vi "Read Drive Operation.vi"(8 "Command Info":T3) -> (0 "Command Info":T3, 1 "SubSystem Data":T1)   [LabVIEW 2017]
doc: "Returns the details about the currently executing command."
uses:
  Implementation/Drive Operations.ctl
  Implementation/Drive Setpoints.ctl
  <vilib>/Rock Robotics/WPI/Framework/Completion Status.ctl
  <vilib>/Rock Robotics/WPI/Framework/Completion Notifier.ctl
  <vilib>/Rock Robotics/WPI/Framework/Command Status Info.ctl
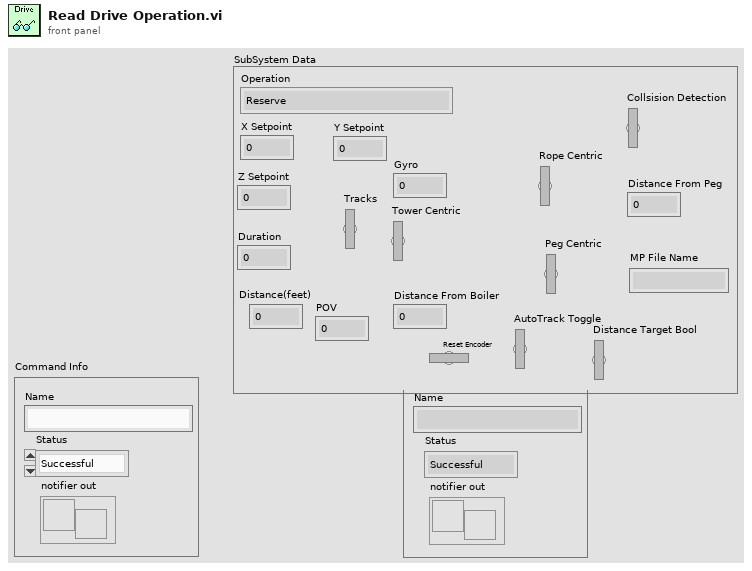
[diagram p1: front panel]
types:
  T1 = typedef "Drive Setpoints.ctl" = cluster{"Operation":T2, "X Setpoint":dbl, "Y Setpoint":dbl, "Duration":dbl, "Z Setpoint":dbl, "Tracks":bool, "Gyro":dbl, "Tower Centric":bool, "POV":i16, "Distance(feet)":dbl, "Distance From Boiler":dbl, "Peg Centric":bool, "Rope Centric":bool, "Distance Target Bool":bool, "AutoTrack Toggle":bool, "Collsision Detection":bool, "Distance From Peg":dbl, "Reset Encoder":bool, "MP File Name":string}
  T2 = typedef "Drive Operations.ctl" = enum16{"Reserve", "Motion Profiling", "Read Current", "Immediate Robot Centric", "Drive for Time Robot Centric", "Immediate Field Centric", "Drive For Time Field Centric", "Immediate MecaTrak", "Drive For Time MecaTrak", "Button Adjust", "Drive for Distance", "Drive Directional Immediate"}
  T3 = typedef "Command Status Info.ctl" = cluster{"Name":string, "Status":T4, "notifier out":T5}
  T4 = typedef "Completion Status.ctl" = enum16{"Successful", "Aborted", "Incomplete"}
  T5 = typedef "Completion Notifier.ctl" = refnum<notifier>
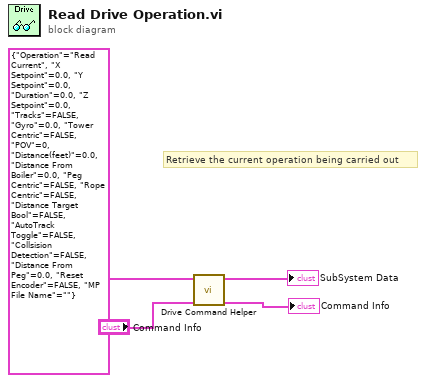
[diagram p0: block diagram]
diagram:
  # "Retrieve the current operation being carried out"
  n1 = call "Drive Command Helper.vi"("Command Info In"="Command Info", "SubSystem Data"=T1 {"Operation"=enum."Read Current", "X Setpoint"=0.0, "Y Setpoint"=0.0, "Duration"=0.0, "Z Setpoint"=0.0, "Tracks"=FALSE, "Gyro"=0.0, "Tower Centric"=FALSE, "POV"=0, "Distance(feet)"=0.0, "Distance From Boiler"=0.0, "Peg Centric"=FALSE, "Rope Centric"=FALSE, "Distance Target Bool"=FALSE, "AutoTrack Toggle"=FALSE, "Collsision Detection"=FALSE, "Distance From Peg"=0.0, "Reset Encoder"=FALSE, "MP File Name"=""}) -> ("Command Info Out"=→"Command Info":T3, "SubSystem Data"=→"SubSystem Data":T1)  [unwired: 8 in]
